vi "FFT算法试验.vi"() -> ()   [LabVIEW 2014]
uses:
  <vilib>/Analysis/2dsp.llb/Real FFT.vi
  <vilib>/Analysis/2dsp.llb/Inverse Real FFT.vi
  <vilib>/express/express analysis/Spectral/Block/exnSpectralBlock spectral measurements peak poly.vi
  <vilib>/express/express analysis/Spectral/Block/exnSpectralBlock spectral measurements peak WFM.vi
  <vilib>/express/express analysis/Spectral/XNode/ExpressSpectralMeasurementsBlockNode.xnode
  <vilib>/measure/NI_MABase.lvlib
  <vilib>/Analysis/NI_AALPro.lvlib
panel:
  in  "滑动杆":dbl(slide) scale=0.0..100.0
  out "滤波后时域信号354":cluster{"f0":dbl, "df":dbl, "magnitude":dbl[]}(graph)
  out "滤波后时域信号35 3":waveform(dbl)(graph)
  in  "样本大小":dbl
  in  "工频频率":dbl
  out "滤波后时域信号36":dbl[](graph)
  out "滤波后时域信号3 5":dbl[](graph)
  out "滤波后时域信号35 2":cluster{"f0":dbl, "df":dbl, "magnitude":dbl[]}(graph)
  out "滤波后时域信号35":waveform(dbl)(graph)
  out "滤波后时域信号3 4":dbl[](graph)
  out "滤波后时域信号34":cluster{"f0":dbl, "df":dbl, "magnitude":dbl[]}(graph)
  out "滤波后时域信号3 3":waveform(dbl)(graph)
  out "滤波后时域信号3 2":dbl[](graph)
  out "滤波后时域信号3":dbl[](graph)
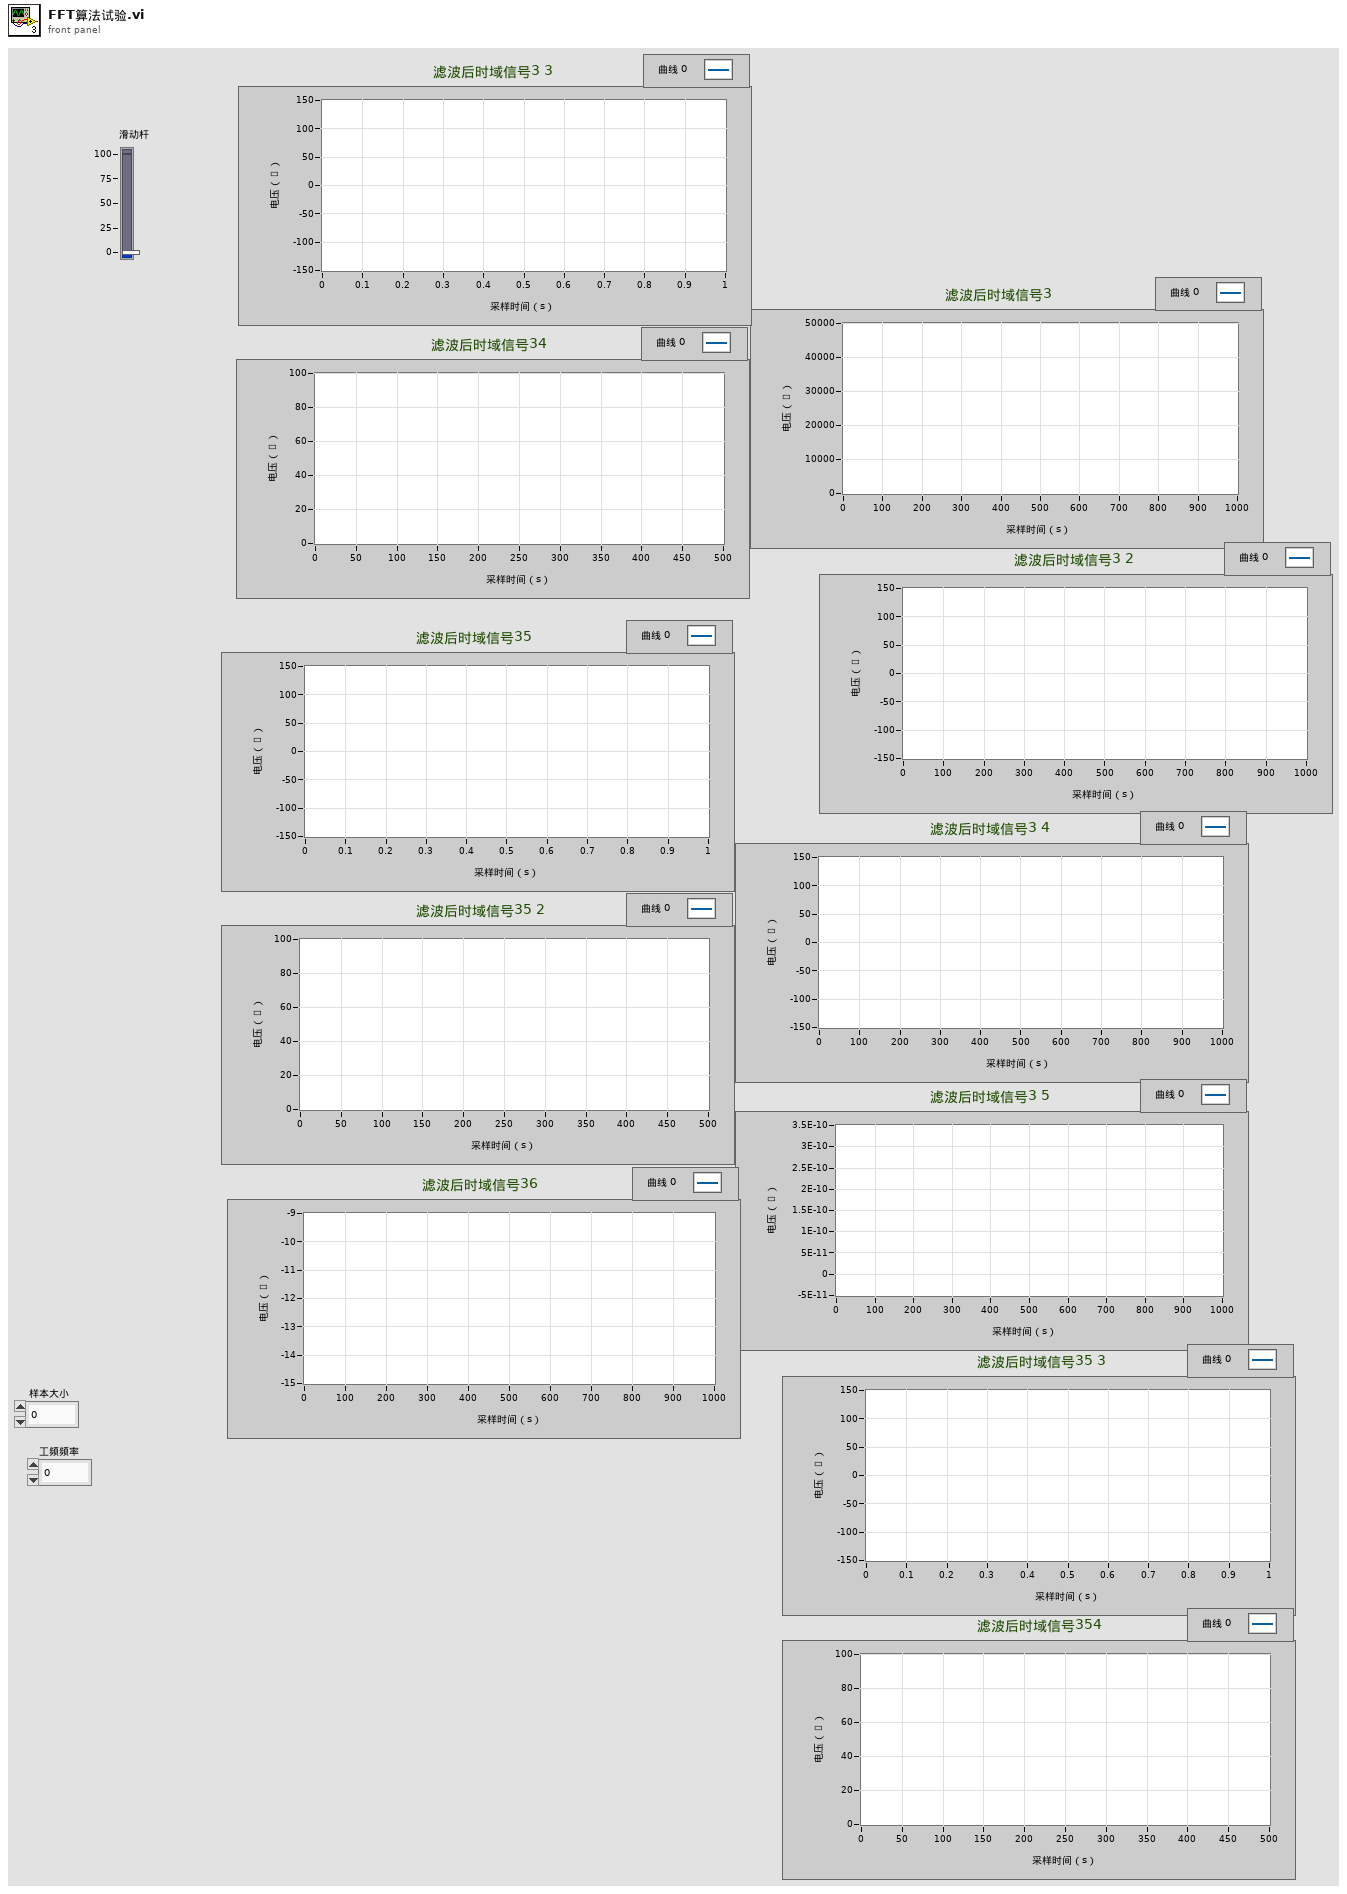
[diagram p1: front panel]
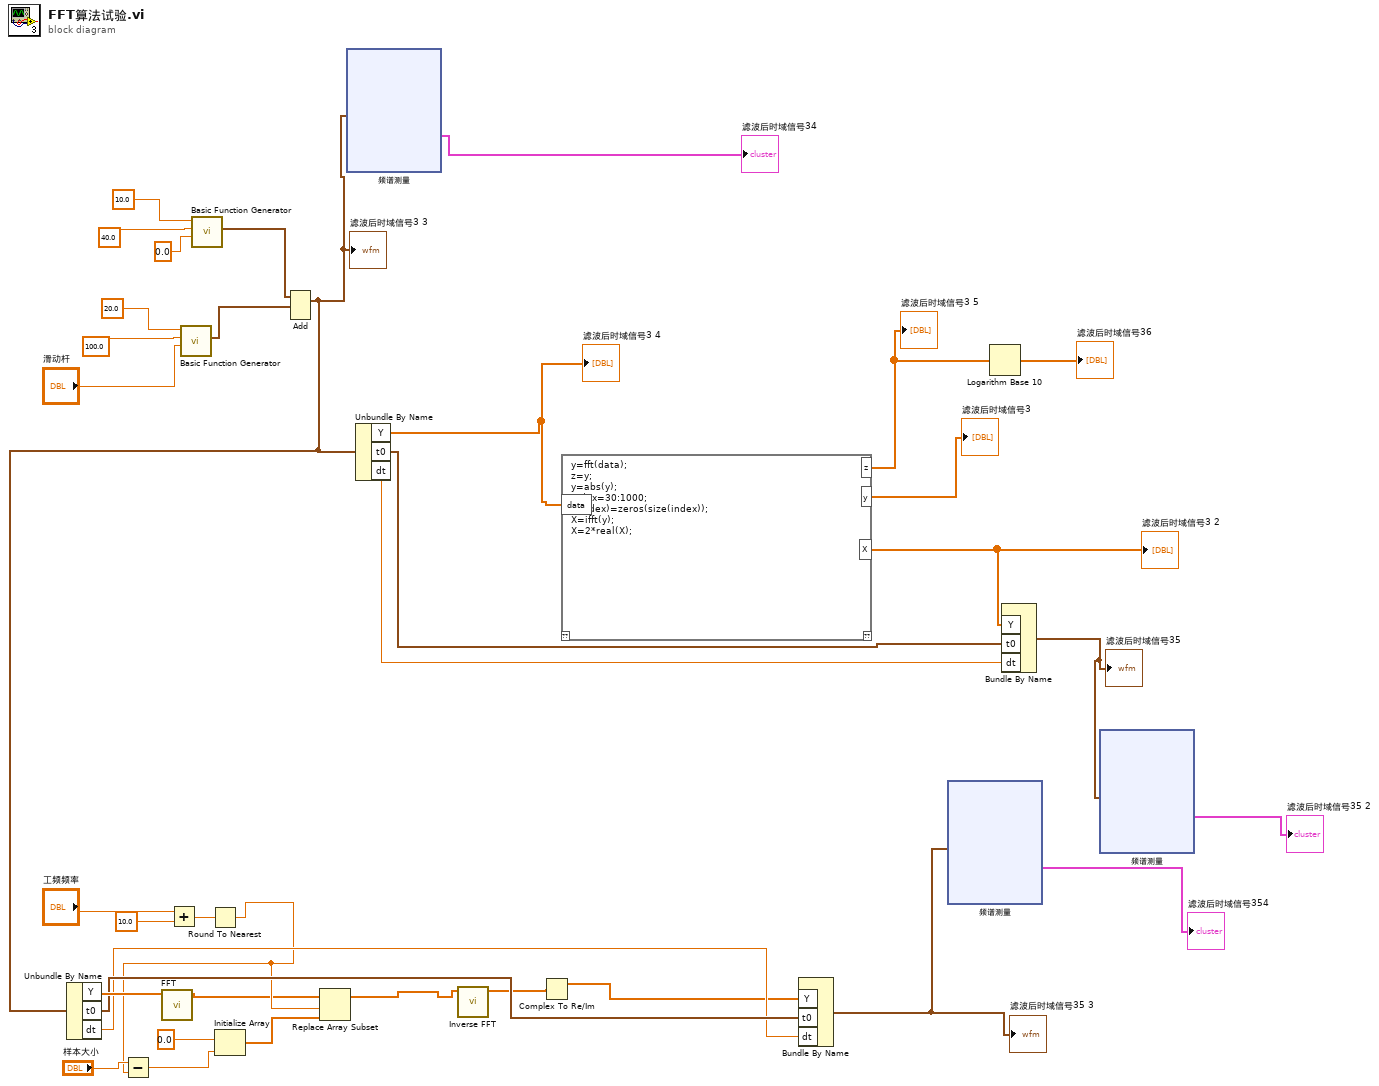
[diagram p0: block diagram]
diagram:
  n1 = Add(x="工频频率", y=10.0) -> (x+y=w14:dbl)
  n2 = call <vilib>:"Basic Function Generator.vi"("phase"="滑动杆", "amplitude"=100.0, "frequency"=20.0) -> ("signal out"=w29:waveform(dbl))  [unwired: 6 in, 2 out]
  n3 = call <vilib>:"Basic Function Generator.vi"("phase"=0.0, "amplitude"=40.0, "frequency"=10.0) -> ("signal out"=w30:waveform(dbl))  [unwired: 6 in, 2 out]
  n4 = Round To Nearest(number=w14) -> (nearest integer value=w8:dbl)
  n5 = Subtract(x="样本大小", y=w8) -> (x-y=w12:dbl)
  n6 = Initialize Array(0.0, w12) -> (w17:dbl[])
  n7 = Add(1:w29, 2:w30) -> (0:w9:waveform(dbl))  [unwired: 1 in, 1 out]
  "滤波后时域信号3 3" <- w9
  n8 = Unbundle By Name(w9) -> ("Y"=w19:dbl[], "t0"=w11:timestamp, "dt"=w10:dbl)
  n9 = call-poly <vilib>:"FFT.vi"("X"=w19) -> ("FFT {X}"=w3:cdb[])  [unwired: 9 in, 1 out]
  n10 = Replace Array Subset(array=w3, new element=w17, index=w8) -> (w5:cdb[])
  n11 = xnode "频谱测量"("信号"=w9) -> ("FFT - （峰值）"=→"滤波后时域信号34":cluster{"f0":dbl, "df":dbl, "magnitude":dbl[]})  [unwired: 1 in, 2 out]
  n12 = Unbundle By Name(w9) -> ("Y"=w27:dbl[], "t0"=w26:timestamp, "dt"=w25:dbl)
  "滤波后时域信号3 4" <- w27
  n13 = call-poly <vilib>:"Inverse FFT.vi"("FFT {X}"=w5) -> ("X"=w2:dbl[])  [unwired: 9 in, 1 out]
  n14 = Complex To Re/Im(x + iy=w2) -> (x=w1:dbl[])  [unwired: 1 out]
  n15 = script code="y=fft(data);\nz=y;\ny=abs(y);\nindex=30:1000;\ny(index)=zeros(size(index));\nX=ifft(y);\nX=2*real(X);"("data"=w27) -> ("y"=→"滤波后时域信号3":dbl[], "X"=w23:dbl[], "z"=w21:dbl[])  [unwired: 1 in, 1 out]
  "滤波后时域信号3 2" <- w23
  "滤波后时域信号3 5" <- w21
  n16 = Bundle By Name("Y"=w1, "t0"=w11, "dt"=w10) -> (w7:waveform(dbl))  [unwired: 1 in]
  "滤波后时域信号35 3" <- w7
  n17 = xnode "频谱测量"("信号"=w7) -> ("FFT - （峰值）"=→"滤波后时域信号354":cluster{"f0":dbl, "df":dbl, "magnitude":dbl[]})  [unwired: 1 in, 2 out]
  n18 = Logarithm Base 10(1:w21) -> (0:→"滤波后时域信号36":dbl[])
  n19 = Bundle By Name("Y"=w23, "t0"=w26, "dt"=w25) -> (w22:waveform(dbl))  [unwired: 1 in]
  "滤波后时域信号35" <- w22
  n20 = xnode "频谱测量"("信号"=w22) -> ("FFT - （峰值）"=→"滤波后时域信号35 2":cluster{"f0":dbl, "df":dbl, "magnitude":dbl[]})  [unwired: 1 in, 2 out]
